vi "Read_XML-File_000.vi"() -> ()   [LabVIEW 2017]
uses:
  D:/MS Project/MS Project/bin/Debug/Ballard_BTI_XML_Deserializer.dll
  MS Project/bin/Debug/Ballard_BTI_XML_Deserializer.dll
panel:
  in  "XML Schema File Path":path=path "\\\\Vboxsvr\\2017/XML Files/BTI.XSD"
  in  "XML Configuration File Path":path=path "\\\\Vboxsvr\\2017/XML Files/XML_000.XML"
  in  "error in (no error)":errorcluster
  out "Array 9":i32[](array[numeric])
  out "Array 8":i32[](array[numeric])
  out "Array 7":string[](array[string])
  out "Array 6":i32[](array[numeric])
  out "Array 5":string[](array[string])
  out "rawData":u8[][](array[numeric])
  out "Array 4":string[](array[string])
  out "Array 2":i32[](array[numeric])
  out "Array":string[](array[string])
  out "error out":errorcluster
  out "name":string
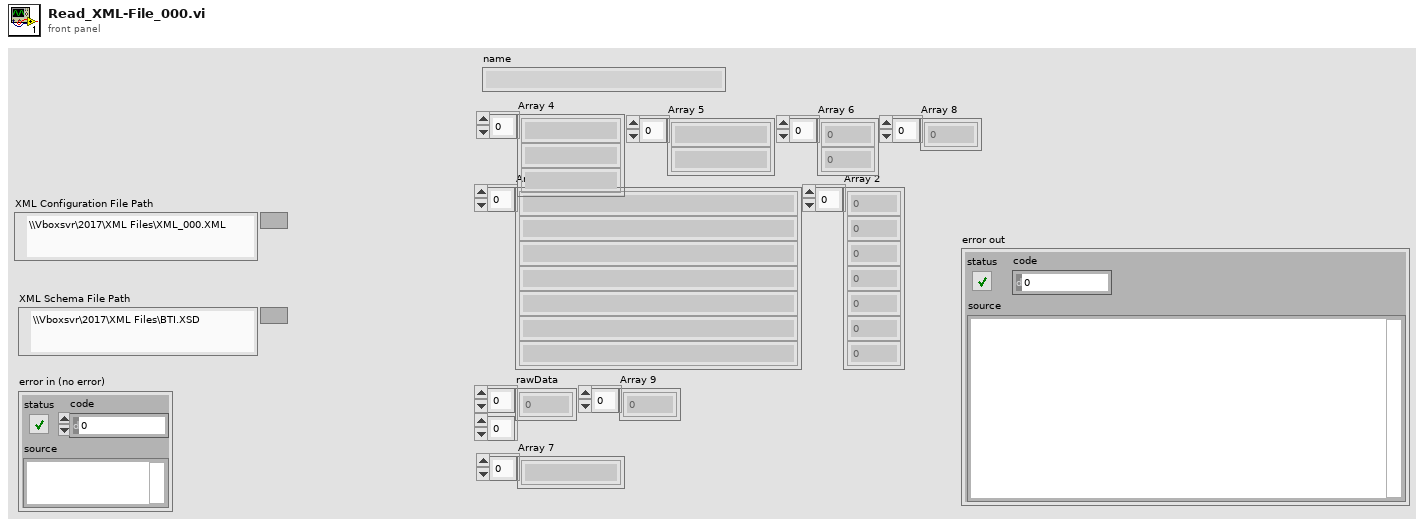
[diagram p1: front panel]
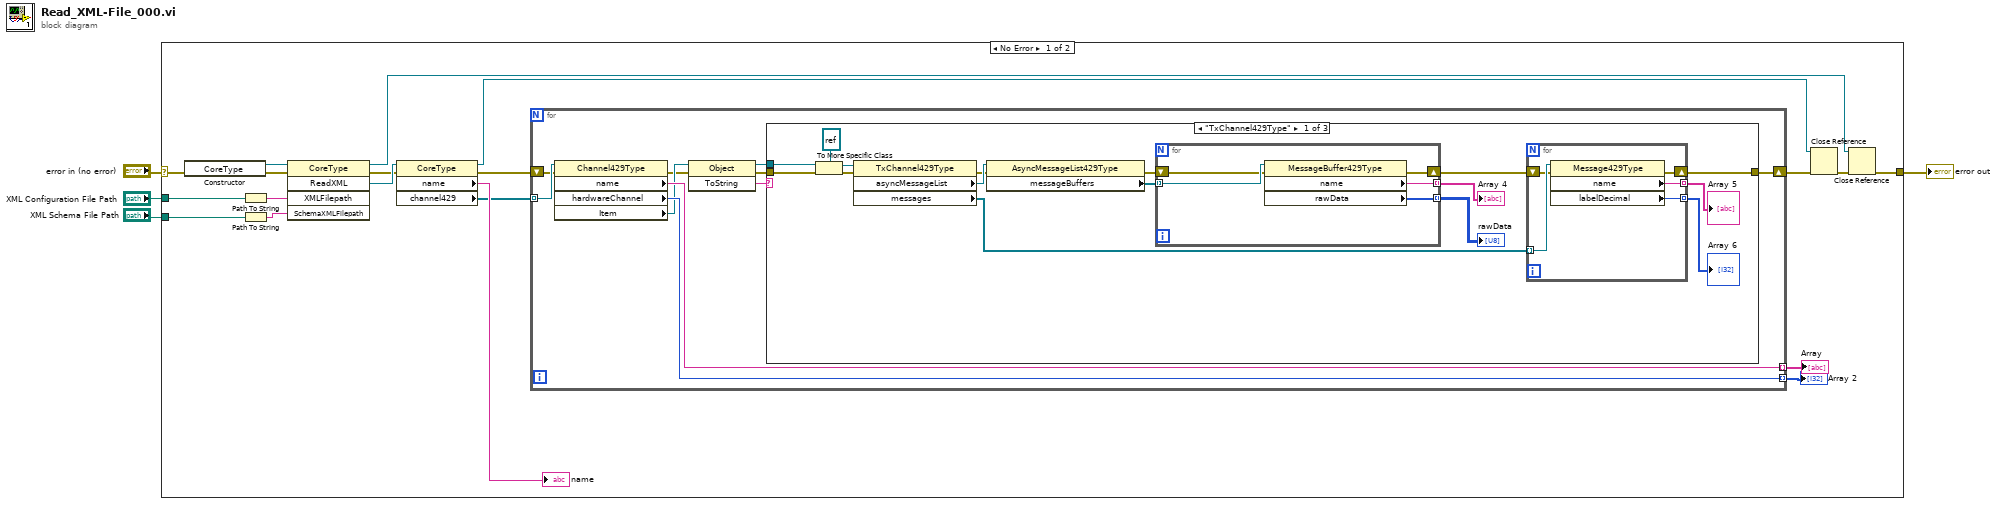
[diagram p0: block diagram]
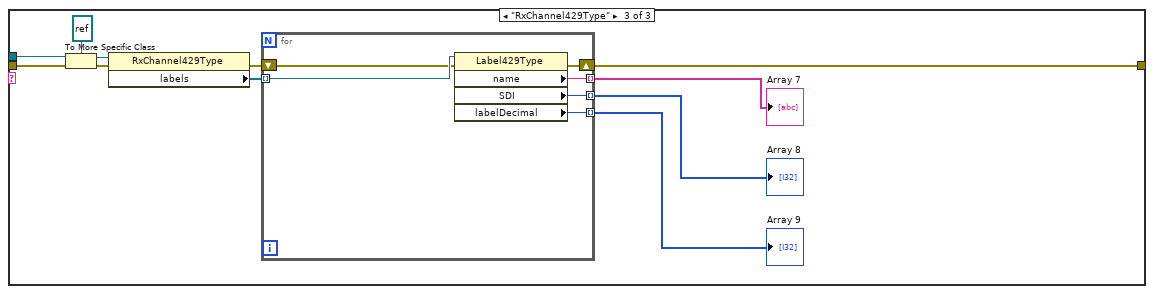
[diagram p3: hidden frame]
diagram:
  n1 = case shown="No Error" "error in (no error)" {
    selector: "error in (no error)" -> [w5 w78]
    tunnel: "XML Configuration File Path" -> [w22 _]
    tunnel: "XML Schema File Path" -> [w14 _]
    tunnel: [w7 w78] -> w2
    frame No Error {
      n2 = constructor class="CoreType"(error in=w5) -> (reference out=w12:refnum<k24>, error out=w11:errorcluster)  [unwired: 2 in, 1 out]
      n3 = Path To String(path=w22) -> (string=w23:string)
      n4 = Path To String(path=w14) -> (string=w13:string)
      n5 = invoke class="CoreType" method="ReadXML"(reference=w12, error in=w11, "XMLFilepath"=w23, "SchemaXMLFilepath"=w13) -> (reference out=w6:refnum<k24>, error out=w20:errorcluster, "ReadXML"=w21:refnum<k24>)  [unwired: 1 in, 2 out]
      n6 = property class="CoreType"(reference=w21, error in=w20) -> (reference out=w9:refnum<k24>, error out=w15:errorcluster, "name"=→"name":string, "channel429"=w18:refnum<k24>[])
      n7 = for {
        tunnel: w18 -> [w31] mode=indexing
        tunnel: [w33] -> w17 mode=indexing
        tunnel: [w32] -> w16 mode=indexing
        shift-right: [w24] -> w10
        shift-left: w15 -> [w27]
        n8 = property class="Channel429Type"(reference=w31, error in=w27) -> (error out=w26:errorcluster, "name"=w33:string, "hardwareChannel"=w32:i32, "Item"=w30:refnum<k24>)  [unwired: 1 out]
        n9 = invoke class="Object" method="ToString"(reference=w30, error in=w26) -> (reference out=w28:refnum<k24>, error out=w25:errorcluster, "ToString"=w29:string)  [unwired: 1 in]
        n10 = case shown="\"TxChannel429Type\"" w29 {
          tunnel: w28 -> [w49 _ w71]
          tunnel: w25 -> [w48 w60 w70]
          tunnel: [w34 w60 w64] -> w24
          frame "TxChannel429Type" {
            n11 = To More Specific Class(target class=refnum<k24> refnum, reference=w49, error in=w48) -> (specific class reference=w45:refnum<k24>, error out=w46:errorcluster)
            n12 = property class="TxChannel429Type"(reference=w45, error in=w46) -> (error out=w43:errorcluster, "asyncMessageList"=w44:refnum<k24>, "messages"=w40:refnum<k24>[])  [unwired: 1 out]
            n13 = property class="AsyncMessageList429Type"(reference=w44, error in=w43) -> (error out=w41:errorcluster, "messageBuffers"=w42:refnum<k24>[])  [unwired: 1 out]
            n14 = for {
              tunnel: w42 -> [w59] mode=indexing
              shift-right: [w57] -> w39
              shift-left: w41 -> [w58]
              tunnel: [w56] -> w38 mode=indexing
              tunnel: [w55] -> w37 mode=indexing
              n15 = property class="MessageBuffer429Type"(reference=w59, error in=w58) -> (error out=w57:errorcluster, "name"=w56:string, "rawData"=w55:u8[])  [unwired: 1 out]
            }
            "Array 4" <- w38
            "rawData" <- w37
            n16 = for {
              tunnel: w40 -> [w54] mode=indexing
              tunnel: [w52] -> w36 mode=indexing
              tunnel: [w51] -> w35 mode=indexing
              shift-right: [w50] -> w34
              shift-left: w39 -> [w53]
              n17 = property class="Message429Type"(reference=w54, error in=w53) -> (error out=w50:errorcluster, "name"=w52:string, "labelDecimal"=w51:i32)  [unwired: 1 out]
            }
            "Array 5" <- w36
            "Array 6" <- w35
          }
          frame "False", Default {
          }
          frame "RxChannel429Type" {
            n18 = To More Specific Class(target class=refnum<k24> refnum, reference=w71, error in=w70) -> (specific class reference=w67:refnum<k24>, error out=w68:errorcluster)
            n19 = property class="RxChannel429Type"(reference=w67, error in=w68) -> (error out=w65:errorcluster, "labels"=w66:refnum<k24>[])  [unwired: 1 out]
            n20 = for {
              tunnel: w66 -> [w77] mode=indexing
              shift-right: [w75] -> w64
              shift-left: w65 -> [w76]
              tunnel: [w74] -> w63 mode=indexing
              tunnel: [w73] -> w62 mode=indexing
              tunnel: [w72] -> w61 mode=indexing
              n21 = property class="Label429Type"(reference=w77, error in=w76) -> (error out=w75:errorcluster, "name"=w74:string, "SDI"=w73:i32, "labelDecimal"=w72:i32)  [unwired: 1 out]
            }
            "Array 7" <- w63
            "Array 8" <- w62
            "Array 9" <- w61
          }
        }
      }
      "Array" <- w17
      "Array 2" <- w16
      n22 = Close Reference(reference=w9, error in (no error)=w10) -> (error out=w8:errorcluster)
      n23 = Close Reference(reference=w6, error in (no error)=w8) -> (error out=w7:errorcluster)
    }
    frame Error {
    }
  }
  "error out" <- w2
